vi "SetAutoGainHeight.vi"(2 "错误输入（无错误）":errorcluster, 3 "自动增益高度百分比":u16) -> (0 "错误输出":errorcluster)   [LabVIEW 2018]
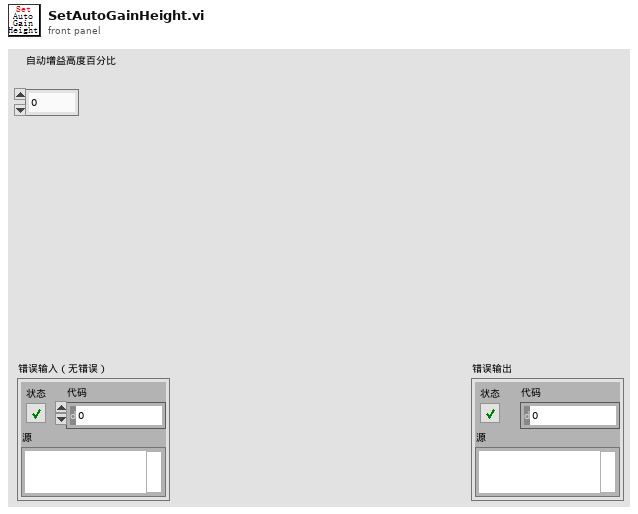
[diagram p1: front panel]
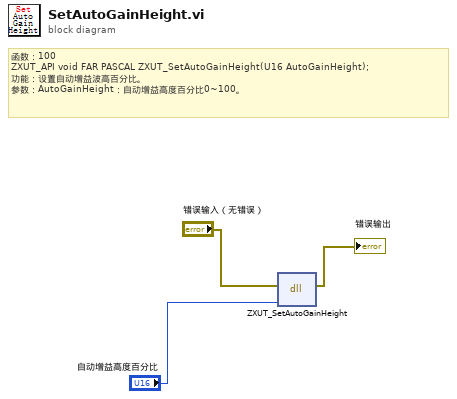
[diagram p0: block diagram]
diagram:
  # "函数：100\nZXUT_API void\tFAR PASCAL ZXUT_SetAutoGainHeight(U16 AutoGainHeight);\n功能：设置自动增益波高百分比。\n参数：AutoGainHeight：自动增益高度百分比0~100。"
  n1 = dll-call lib="PTH2Rabs E软件项目超声超声子VI函数VI\tTCG处理ZXUTConfigMgr.dll" fn="ZXUT_SetAutoGainHeight"(error in="错误输入（无错误）", "AutoGainHeight"="自动增益高度百分比") -> (error out=→"错误输出":errorcluster)  [unwired: 4 in, 1 out]
